vi "CreateInterface.vi"(0 "ClassWriterNative.lvclass":refnum<class "ClassWriterNative.lvclass">, 1 "ProjectTreePosition(String or Project Item Ref)":variant, 2 "CreateInterfaceData":T1, 5 "error in (no error)":errorcluster, 6 "KeepLvClassRefOpen(False)":bool, 7 "HeaderToApply (take from VIRef or /use 2D-8bit header, Ignored if not wired)":variant) -> (14 "ClassWriterNative.lvclass":refnum<class "ClassWriterNative.lvclass">, 15 "LVClassLibraryRefnum":refnum<vi>, 19 "error out":errorcluster)   [LabVIEW 2020, in "ClassWriterNative.lvclass"]
uses:
  <resource>/Framework/Providers/Open_GDS/ClassProviders/Provider_LvNativeClass/ClassWriterNative_class/ClassWriterNative.lvclass
  <resource>/Framework/Providers/Open_GDS/ClassProviders/Provider_BaseClassInterface/CreateInterfaceData.ctl
  <resource>/Framework/Providers/Open_GDS/ClassProviders/Provider_BaseClassInterface/ClassWriter_class/InterfaceMethodsToCreate.ctl
  <resource>/Framework/Providers/Open_GDS/ClassProviders/Common/CommonVIs/CommonVIs_AttributeType.ctl
  <resource>/Framework/Providers/Open_GDS/ClassProviders/Common/CommonVIs/CommonVIs_AttributeDataType.ctl
  <resource>/Framework/Providers/Open_GDS/ClassProviders/Common/String/GDSString_AccessScopeModifierType.ctl
  <resource>/Framework/Providers/Open_GDS/ClassProviders/Common/LvClass_class/GDSLvCLass_ClassSettingsType.ctl
  <resource>/Framework/Providers/Open_GDS/ClassProviders/Common/LvClass_class/GDSLvClass_PlugIn.ctl
  <resource>/Framework/Providers/Open_GDS/ClassProviders/Common/LvClass_class/GDSLvClass_PlugInTypes.ctl
  <resource>/Framework/Providers/Open_GDS/ClassProviders/Provider_LvNativeClass/LvNativeProviderName.ctl
  <resource>/Framework/Providers/Open_GDS/ClassProviders/Provider_BaseClassInterface/ClassApperanceType.ctl
  <resource>/Framework/Providers/Open_GDS/API/GDSAPI_SubVIs/GDSAPI_MethodType.ctl
  <resource>/Framework/Providers/Open_GDS/ClassProviders/Provider_BaseClassInterface/CreateMethodData.ctl
  <resource>/Framework/Providers/Open_GDS/ClassProviders/Provider_EndevoGOOP300/GOOP300_SubVIs/GOOP300_MethodScopeType.ctl
  <resource>/Framework/Providers/Open_GDS/ClassProviders/Provider_LvNativeClass/ClassWriterNative_class/IconDetails.ctl
  <resource>/Framework/Providers/Open_GDS/ClassProviders/Provider_LvNativeClass/ClassWriterNative_class/IconSize.ctl
  <resource>/Framework/Providers/Open_GDS/ClassProviders/Common/InterfaceLibrary/InterfaceLibrary.lvlib
  <resource>/Framework/Providers/Open_GDS/ClassProviders/Provider_BaseClassInterface/ClassWriter_class/ClassWriter.lvclass
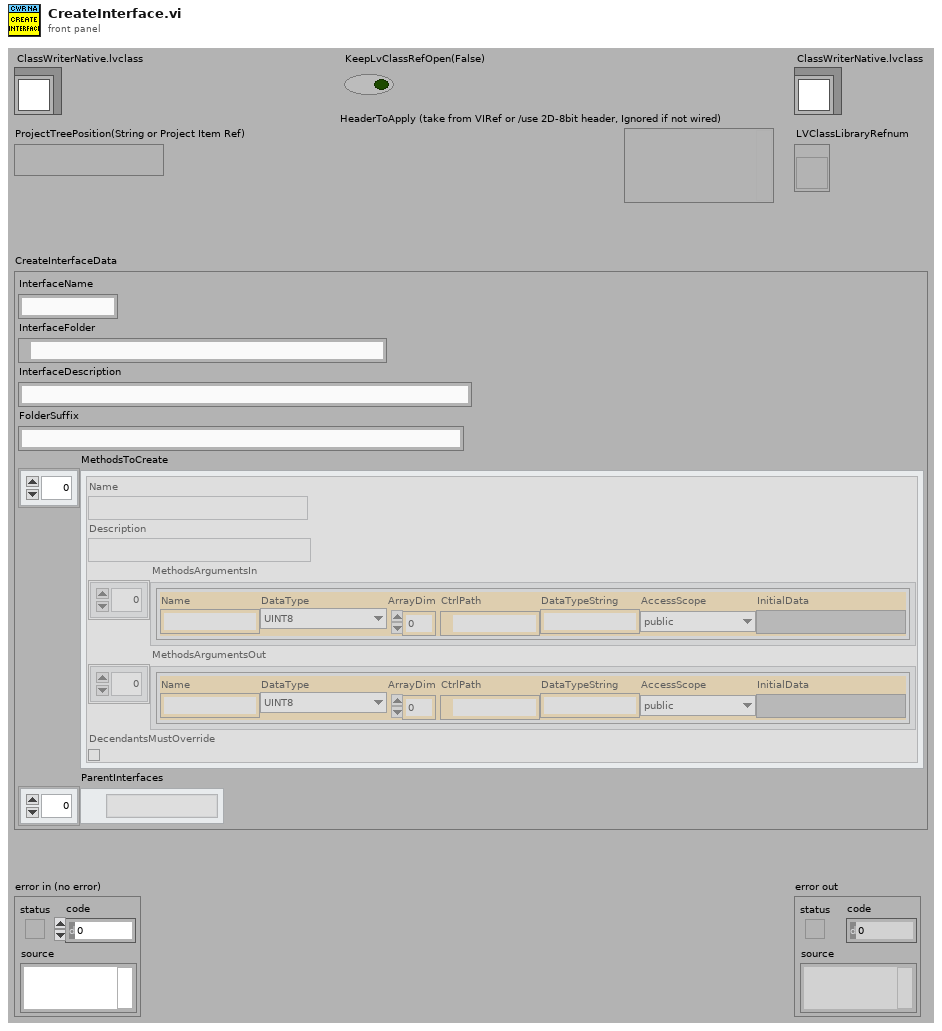
[diagram p1: front panel]
types:
  T1 = typedef "ClassWriter.lvclass/CreateInterfaceData.ctl" = cluster{"InterfaceName":string, "InterfaceFolder":path, "InterfaceDescription":string, "FolderSuffix":string, "MethodsToCreate":T2[], "ParentInterfaces":path[]}
  T2 = typedef "ClassWriter.lvclass/InterfaceMethodsToCreate.ctl" = cluster{"Name":string, "Description":string, "MethodsArgumentsIn":T3[], "MethodsArgumentsOut":T3[], "DecendantsMustOverride":bool}
  T3 = typedef "CommonVIs_AttributeType.ctl" = cluster{"Name":string, "DataType":T4, "ArrayDim":i32, "CtrlPath":path, "DataTypeString":string, "AccessScope":T5, "InitialData":variant}
  T4 = typedef "CommonVIs_AttributeDataType.ctl" = enum16{"UINT8", "INT8", "UINT16", "INT16", "UINT32", "INT32", "UINT64", "INT64", "SGL", "DBL", "EXT", "CSG", "CDB", "CXT", "TimeStamp", "STRING", "PATH", "BOOL", "ENUM", "RefNum", "VIRefNum", "LabVIEW Class", "Cluster", "Variant", "TypeDef", "Waveform", "LabVIEW Object", "Other", "void", "Set", "Map"}
  T5 = typedef "GDSString_AccessScopeModifierType.ctl" = enum16{"public", "private", "protected", "internal"}
  T6 = cluster{"InterfacePath":path, "InterfaceRefnum":refnum<vi>, "ProjectRefnum":refnum<vi>, "LvClassFolderPath":path, "App":refnum<vi>, "Project Item":refnum<vi>, "InterfaceName":string, "ProjectItemIn":bool}
  T7 = typedef "ClassApperanceType.ctl" = enum16{"Class", "AF-MessageClass", "Interface"}
  T8 = typedef "LvNativeProviderName.ctl" = enum16{"Endevo LabVIEW Native"}
  T9 = typedef "GDSLvCLass_ClassSettingsType.ctl" = cluster{"ClassProviderName":string, "ClassTemplateUsed":string, "ClassTemplateVersion":string, "ClassDescription":string, "PlugIns":T10[], "ConnectorPanePattern":string}
  T10 = typedef "GDSLvClass_PlugIn.ctl" = cluster{"Type":T11, "ID":string, "Version":string, "Path":path, "Name":string, "Data":variant}
  T11 = typedef "GDSLvClass_PlugInTypes.ctl" = enum16{"DesignPattern", "MethodTypes"}
  T12 = typedef "GDSAPI_MethodType.ctl" = enum16{"Read Attribute", "Write Attribute", "Read & Write Attribute", "None Modifying Method", "Get Property", "Set Property", "Read Property", "Write Property", "Static Method", "Interface Method"}
  T13 = typedef "GOOP300_MethodScopeType.ctl" = enum16{"Use Parent Folder Scope", "Public", "Protected", "Private", "Community"}
  T14 = typedef "ClassWriter.lvclass/CreateMethodData.ctl" = cluster{"MethodName":string, "RelativeMethodPath":path, "MethodDescription":string, "Scope/Visibility":T13, "MethodTemplateName":string, "IconOut":u8[][], "RelativeProjectClassPath":string, "OpenViAfterCreation":bool, "DynamicDispatchVi":bool, "ExtraCreateParameters":variant, "MustOverride":bool, "MustCallParent":bool, "IconDetails":T15, "AF-Option":variant, "TemplatePath":path}
  T15 = typedef "ClassWriterNative.lvclass/IconDetails.ctl" = cluster{"IconSize":T16, "ImageRows(32)":i32, "ConnectorPaneHeight":i32[]}
  T16 = typedef "ClassWriterNative.lvclass/IconSize.ctl" = enum16{"Full", "1 c-term high", "2 c-term high", "3 c-term high"}
  T17 = typedef "Scripting_ConnectorPanePatternType.ctl" = u16
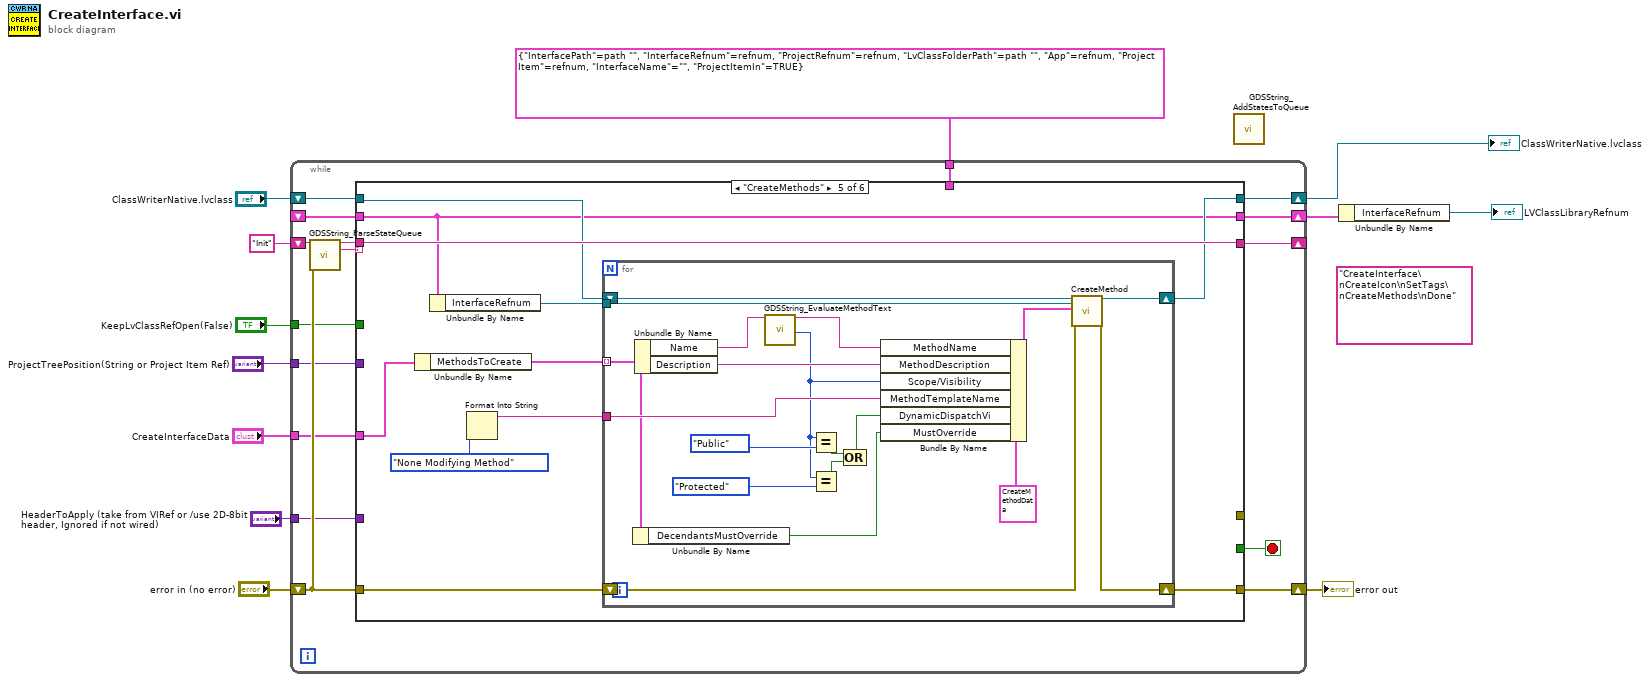
[diagram p0: block diagram]
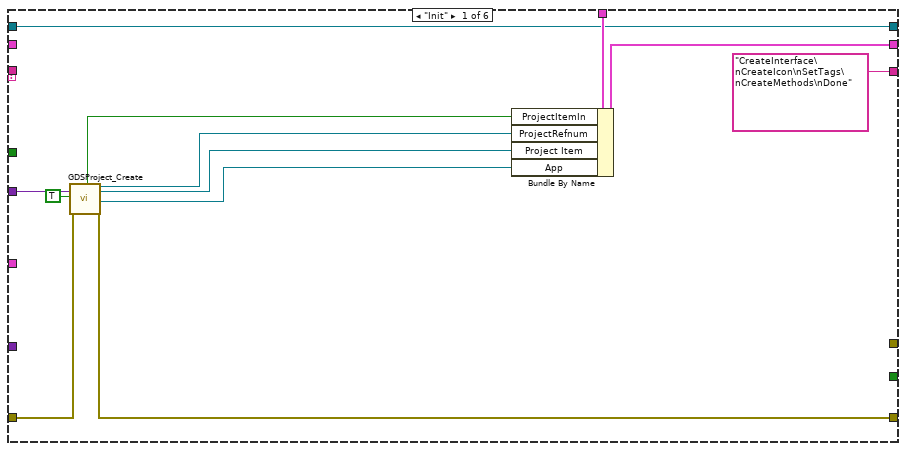
[diagram p2: hidden frame]
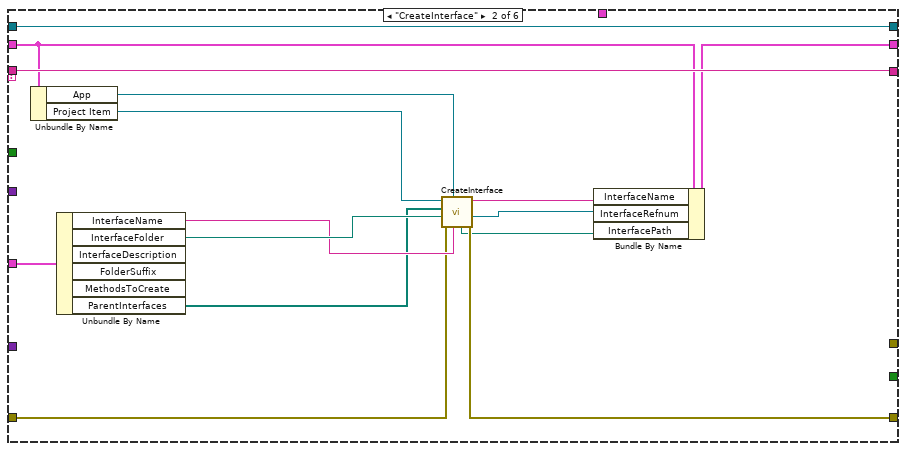
[diagram p3: hidden frame]
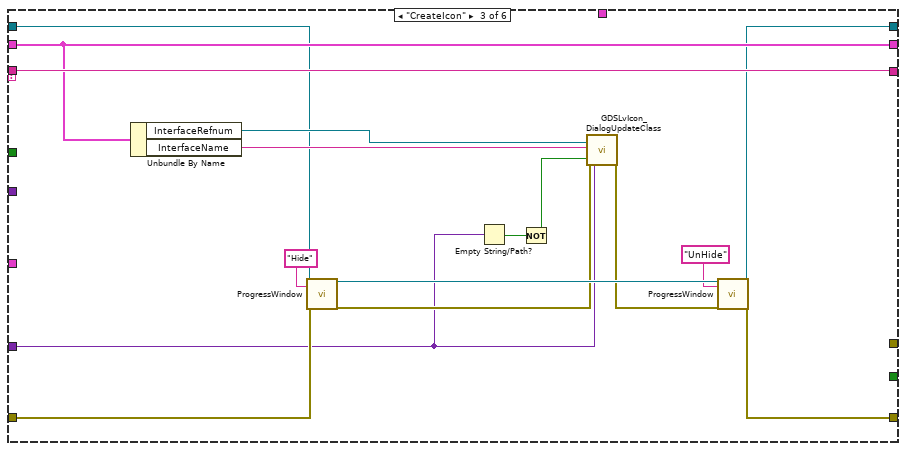
[diagram p4: hidden frame]
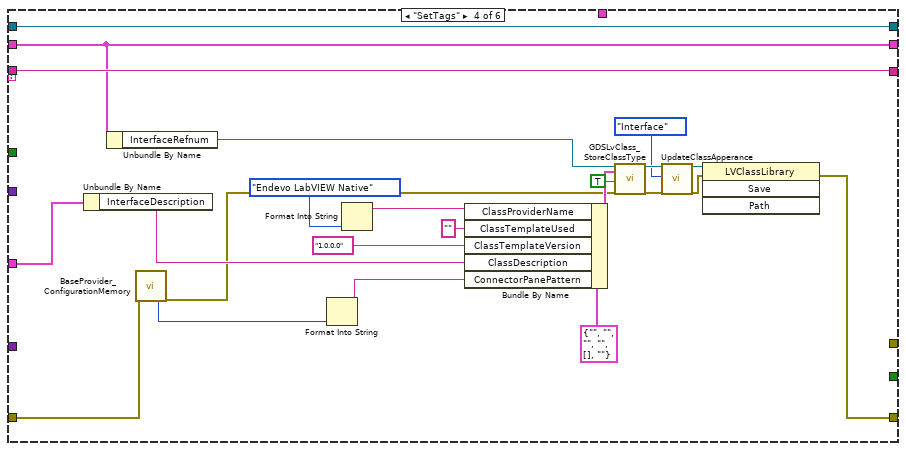
[diagram p5: hidden frame]
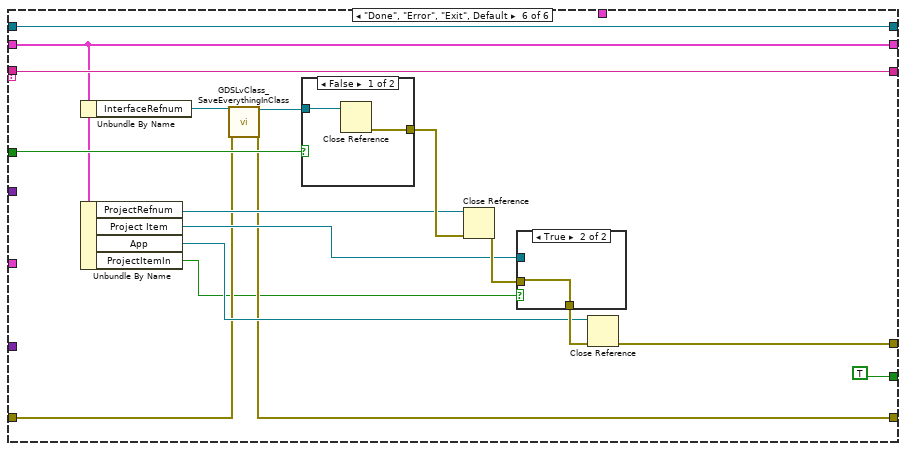
[diagram p6: hidden frame]
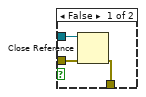
[diagram p7: hidden frame]
diagram:
  (unwired) "CreateInterface\nCreateIcon\nSetTags\nCreateMethods\nDone"
  n1 = while {
    shift-right: [w25] -> _
    shift-left: "Init" -> [w27]
    shift-right: [w23] -> w3
    shift-left: "error in (no error)" -> [w24]
    tunnel: "CreateInterfaceData" -> [w22]
    tunnel: T6 {"InterfacePath"=path "", "InterfaceRefnum"=refnum, "ProjectRefnum"=refnum, "LvClassFolderPath"=path "", "App"=refnum, "Project Item"=refnum, "InterfaceName"="", "ProjectItemIn"=TRUE} ("output cluster") -> [w21]
    shift-right: [w20] -> w6
    shift-left: _ -> [w19]
    tunnel: "ProjectTreePosition(String or Project Item Ref)" -> [w18]
    tunnel: "HeaderToApply (take from VIRef or /use 2D-8bit header, Ignored if not wired)" -> [w17]
    tunnel: "KeepLvClassRefOpen(False)" -> [w16]
    shift-right: [w13] -> w1
    shift-left: "ClassWriterNative.lvclass" -> [w14]
    stop <- w15 stop-if-true
    n2 = call <resource>:"GDSString_ParseStateQueue.vi"("State Queue"=w27, "Error In (no error)"=w24) -> ("Remaining States"=w26:string, "Current State"=w28:string)  [unwired: 9 in, 3 out]
    n3 = case shown="\"CreateMethods\"" w28 {
      tunnel: ["CreateInterface\nCreateIcon\nSetTags\nCreateMethods\nDone" w55 w71 w94 w105 w141] -> w25
      tunnel: w26 -> [_ w55 w71 w94 w105 w141]
      tunnel: [w33 w49 w63 w76 w102 w127] -> w23
      tunnel: w24 -> [w32 w48 w62 w75 w101 w126]
      tunnel: w22 -> [_ w54 _ w82 w100 _]
      tunnel: w21 -> [w38 _ _ _ _ _]
      tunnel: [w37 w47 w60 w93 w96 w138] -> w20
      tunnel: w19 -> [_ w53 w60 w93 w96 w138]
      tunnel: w18 -> [w39 _ _ _ _ _]
      tunnel: w17 -> [_ _ w61 _ _ _]
      tunnel: w16 -> [_ _ _ _ _ w140]
      tunnel: w14 -> [w30 w42 w56 w73 w103 w130]
      tunnel: [_ _ _ _ _ TRUE] -> w15
      tunnel: [_ _ _ _ _ w131] -> _
      tunnel: [w30 w42 w57 w73 w104 w130] -> w13
      frame "Init" {
        n4 = call <resource>:"GDSProject_Create.vi"("ProjectTreePosition(String or Project Item Ref)"=w39, "AllowPopUpDilaog(True)"=TRUE, "error in (no error)"=w32) -> ("ProjectItemIn"=w29:bool, "Project Refnum"=w35:refnum<vi>, "Project Item"=w34:refnum<vi>, "App"=w36:refnum<vi>, "error out"=w33:errorcluster)  [unwired: 12 in]
        n5 = Bundle By Name(cluster=w38, "ProjectItemIn"=w29, "ProjectRefnum"=w35, "Project Item"=w34, "App"=w36) -> (w37:T6)
      }
      frame "CreateInterface" {
        n6 = Unbundle By Name(w53) -> ("App"=w52:refnum<vi>, "Project Item"=w43:refnum<vi>)
        n7 = Unbundle By Name(w54) -> ("InterfaceName"=w50:string, "InterfaceFolder"=w51:path, "ParentInterfaces"=w41:path[])  [unwired: 3 out]
        n8 = call <resource>:"CreateInterface.vi"("InterfaceName"=w50, "Application"=w52, "error in"=w48, "Interface Folder"=w51, "Parent Interfaces(ClassRef/Path)"=w41, "New Interface Owner"=w43) -> ("error out"=w49:errorcluster, "Interface"=w45:refnum<vi>, "InterfaceName(Non Qualified)"=w46:string, "InterfacePath"=w44:path)  [unwired: 1 in, 1 out]
        n9 = Bundle By Name(cluster=w53, "InterfaceName"=w46, "InterfaceRefnum"=w45, "InterfacePath"=w44) -> (w47:T6)
      }
      frame "CreateIcon" {
        n10 = Unbundle By Name(w60) -> ("InterfaceRefnum"=w58:refnum<vi>, "InterfaceName"=w59:string)
        n11 = call-dynamic "ProgressWindow.vi"("ClassWriter in"=w56, "Message(Exit)"="Hide", "error in (no error)"=w62) -> ("ClassWriter out"=w67:refnum<class "ClassWriterNative.lvclass">, "error out"=w65:errorcluster)  [unwired: 15 in]
        n12 = Empty String/Path?(string/path=w61) -> (empty?=w70:bool)
        n13 = Not(x=w70) -> (.not. x?=w69:bool)
        n14 = call <resource>:"GDSLvIcon_DialogUpdateClass.vi"("ClassPath(FilePath/ProjectTreePath/LvCLassRef)"=w58, "ClassName"=w59, "AutoUpdate"=w69, "error in (no error)"=w65, "HeaderToApply (take from VIRef or /use 2D-8bit header, Ignored if not wired)"=w61) -> ("error out"=w64:errorcluster)  [unwired: 11 in, 3 out]
        n15 = call-dynamic "ProgressWindow.vi"("ClassWriter in"=w67, "Message(Exit)"="UnHide", "error in (no error)"=w64) -> ("ClassWriter out"=w57:refnum<class "ClassWriterNative.lvclass">, "error out"=w63:errorcluster)  [unwired: 15 in]
      }
      frame "SetTags" {
        n16 = Unbundle By Name(w82) -> ("InterfaceDescription"=w81:string)
        n17 = Unbundle By Name(w93) -> ("InterfaceRefnum"=w74:refnum<vi>)
        n18 = call <resource>:"BaseProvider_ConfigurationMemory.vi"("error in (no error)"=w75) -> ("PatternOut"=w84:T17, "error out"=w77:errorcluster)  [unwired: 12 in, 5 out]
        n19 = Format Into String(w84) -> (resulting string=w83:string)  [unwired: 3 in, 1 out]
        n20 = Format Into String(LvNativeProviderName."Endevo LabVIEW Native" ("ProviderName")) -> (resulting string=w79:string)  [unwired: 3 in, 1 out]
        n21 = Bundle By Name(cluster=T9 {"ClassProviderName"="", "ClassTemplateUsed"="", "ClassTemplateVersion"="", "ClassDescription"="", "PlugIns"=[], "ConnectorPanePattern"=""} ("ClassSettings"), "ClassProviderName"=w79, "ClassTemplateUsed"="", "ClassTemplateVersion"="1.0.0.0", "ClassDescription"=w81, "ConnectorPanePattern"=w83) -> (w86:T9)
        n22 = call <resource>:"GDSLvClass_StoreClassType.vi"("Class Refnum In"=w74, "ClassSettings"=w86, "CheckAndFixConnectorPaneType(False)"=TRUE, "error in (no error)"=w77) -> ("Class Refnum Out"=w87:refnum<vi>, "error out"=w88:errorcluster)  [unwired: 14 in]
        n23 = call <resource>:"UpdateClassApperance.vi"("ClassRefIn"=w87, "ClassType(Class)"=ClassApperanceType."Interface", "error in (no error)"=w88) -> ("ClassRefOut"=w89:refnum<vi>, "error out"=w90:errorcluster)  [unwired: 15 in]
        n24 = invoke class="LVClassLibrary" method="Save"(reference=w89, error in=w90) -> (error out=w76:errorcluster)  [unwired: 2 in, 3 out]
      }
      frame "CreateMethods" {
        n25 = Unbundle By Name(w100) -> ("MethodsToCreate"=w97:T2[])
        n26 = Unbundle By Name(w96) -> ("InterfaceRefnum"=w95:refnum<vi>)
        n27 = Format Into String(GDSAPI_MethodType."None Modifying Method" ("MethodType")) -> (resulting string=w98:string)  [unwired: 3 in, 1 out]
        n28 = for {
          shift-right: [w124] -> w104
          shift-left: w103 -> [w123]
          shift-right: [w122] -> w102
          shift-left: w101 -> [w121]
          tunnel: w98 -> [w119]
          tunnel: w97 -> [w107] mode=indexing
          tunnel: w95 -> [w108]
          n29 = Unbundle By Name(w107) -> ("DecendantsMustOverride"=w106:bool)
          n30 = Unbundle By Name(w107) -> ("Name"=w117:string, "Description"=w118:string)
          n31 = call <resource>:"GDSString_EvaluateMethodText.vi"("MethodString"=w117) -> ("MethodName"=w116:string, "Scope/Visibility"=w114:T13)  [unwired: 13 in, 4 out]
          n32 = Equal?(x=w114, y=GOOP300_MethodScopeType."Public" ("Scope/Visibility")) -> (x = y?=w112:bool)
          n33 = Equal?(x=w114, y=GOOP300_MethodScopeType."Protected" ("Scope/Visibility")) -> (x = y?=w111:bool)
          n34 = Compound Arithmetic op=OR(w112, w111) -> (w110:bool)
          n35 = Bundle By Name(cluster=T14 {"MethodName"="", "RelativeMethodPath"=path "", "MethodDescription"="", "Scope/Visibility"=enum."Use Parent Folder Scope", "MethodTemplateName"="", "IconOut"=[], "RelativeProjectClassPath"="", "OpenViAfterCreation"=FALSE, "DynamicDispatchVi"=FALSE, "ExtraCreateParameters"=variant, "MustOverride"=FALSE, "MustCallParent"=FALSE, "IconDetails"={"IconSize"=enum."Full", "ImageRows(32)"=0, "ConnectorPaneHeight"=[]}, "AF-Option"=variant, "TemplatePath"=path ""} ("CreateMethodData"), "MethodName"=w116, "MethodDescription"=w118, "Scope/Visibility"=w114, "MethodTemplateName"=w119, "DynamicDispatchVi"=w110, "MustOverride"=w106) -> (w109:T14)
          n36 = call-dynamic "CreateMethod.vi"("ClassWriterNative.lvclass"=w123, "ClassItemRefIn"=w108, "CreateMethodData"=w109, "error in (no error)"=w121) -> ("ClassWriterNative.lvclass 2"=w124:refnum<class "ClassWriterNative.lvclass">, "error out"=w122:errorcluster)  [unwired: 12 in, 2 out]
        }
      }
      frame "Done", "Error", "Exit", Default {
        n37 = Unbundle By Name(w138) -> ("InterfaceRefnum"=w129:refnum<vi>)
        n38 = Unbundle By Name(w138) -> ("ProjectRefnum"=w136:refnum<vi>, "Project Item"=w134:refnum<vi>, "App"=w132:refnum<vi>, "ProjectItemIn"=w125:bool)
        n39 = call <resource>:"GDSLvClass_SaveEverythingInClass.vi"("ClassRefIn"=w129, "error in"=w126) -> ("ClassRefOut"=w128:refnum<vi>, "error out"=w127:errorcluster)  [unwired: 16 in]
        n40 = case shown="False" w140 {
          tunnel: w128 -> [w147 _]
          tunnel: [w146 _] -> w137
          frame False {
            n41 = Close Reference(reference=w147) -> (error out=w146:errorcluster)  [unwired: 1 in]
          }
          frame True {
          }
        }
        n42 = Close Reference(reference=w136, error in (no error)=w137) -> (error out=w135:errorcluster)
        n43 = case shown="True" w125 {
          tunnel: w135 -> [w144 w145]
          tunnel: w134 -> [w143 _]
          tunnel: [w142 w145] -> w133
          frame False {
            n44 = Close Reference(reference=w143, error in (no error)=w144) -> (error out=w142:errorcluster)
          }
          frame True {
          }
        }
        n45 = Close Reference(reference=w132, error in (no error)=w133) -> (error out=w131:errorcluster)
      }
    }
  }
  "ClassWriterNative.lvclass" <- w1
  "error out" <- w3
  n46 = call <resource>:"GDSString_AddStatesToQueue.vi"() -> ()  [unwired: 15 in, 1 out]
  n47 = Unbundle By Name(w6) -> ("InterfaceRefnum"=→"LVClassLibraryRefnum":refnum<vi>)
